vi "Insert SET ID Signal.vi"(10 "Digital Waveform Graph":digitalwaveform(graph)={"t0"=timestamp(3403282811.6192408 s since 1904-01-01), "dt"=9.615384615384615e-09, "Y"={"transitions"=[], "data"=[[1, 0, 1, 0], [1, 0, 1, 0], [1, 0, 1, 0], [1, 0, 1, 0], [1, 0, 1, 0], [1, 0, 1, 0], [1, 0, 1, 0], [0, 0, 1, 0], [0, 0, 0, 0], [0, 0, 0, 0], [0, 0, 0, 0], [0, 0, 0, 0], [0, 0, 0, 0], [0, 0, 0, 0], [0, 0, 0, 0], [1, 1, 0, 0], [1, 1, 1, 1], [1, 1, 1, 1], [1, 1, 1, 1], [1, 0, 1, 1], [1, 0, 1, 0], [1, 0, 1, 0], [1, 0, 1, 0], [1, 1, 1, 0], [1, 1, 1, 1], [1, 1, 1, 1], [1, 1, 1, 1], [1, 0, 1, 1], [1, 0, 1, 0], [1, 0, 1, 0], [1, 0, 1, 0], [1, 1, 1, 0], [1, 1, 1, 1], [1, 1, 1, 1], [1, 1, 1, 1], [1, 0, 1, 1], [1, 0, 1, 0], [1, 0, 1, 0], [1, 0, 1, 0], [1, 1, 1, 0], [1, 1, 1, 1], [1, 1, 1, 1], [1, 1, 1, 1], [1, 0, 1, 1], [1, 0, 1, 0], [1, 0, 1, 0], [1, 0, 1, 0], [0, 1, 1, 0], [0, 1, 0, 1], [0, 1, 0, 1], [0, 1, 0, 1], [0, 0, 0, 1], [0, 0, 0, 0], [0, 0, 0, 0], [0, 0, 0, 0], [1, 1, 0, 0], [1, 1, 1, 1], [1, 1, 1, 1], [1, 1, 1, 1], [1, 0, 1, 1], [1, 0, 1, 0], [1, 0, 1, 0], [1, 0, 1, 0], [0, 1, 1, 0], [0, 1, 0, 1], [0, 1, 0, 1], [0, 1, 0, 1], [0, 0, 0, 1], [0, 0, 0, 0], [0, 0, 0, 0], [0, 0, 0, 0], [1, 1, 0, 0], [1, 1, 1, 1], [1, 1, 1, 1], [1, 1, 1, 1], [1, 0, 1, 1], [1, 0, 1, 0], [1, 0, 1, 0], [1, 0, 1, 0], [1, 1, 1, 0], [1, 1, 1, 1], [1, 1, 1, 1], [1, 1, 1, 1], [1, 0, 1, 1], [1, 0, 1, 0], [1, 0, 1, 0], [1, 0, 1, 0], [0, 1, 1, 0], [0, 1, 0, 1], [0, 1, 0, 1], [0, 1, 0, 1], [0, 0, 0, 1], [0, 0, 0, 0], [0, 0, 0, 0], [0, 0, 0, 0], [1, 1, 0, 0], [1, 1, 1, 1], [1, 1, 1, 1], [1, 1, 1, 1], [1, 0, 1, 1], [1, 0, 1, 0], [1, 0, 1, 0], [1, 0, 1, 0], [0, 1, 1, 0], [0, 1, 0, 1], [0, 1, 0, 1], [0, 1, 0, 1], [0, 0, 0, 1], [0, 0, 0, 0], [0, 0, 0, 0], [0, 0, 0, 0], [1, 1, 0, 0], [1, 1, 1, 1], [1, 1, 1, 1], [1, 1, 1, 1], [1, 0, 1, 1], [1, 0, 1, 0], [1, 0, 1, 0], [1, 0, 1, 0], [0, 1, 1, 0], [0, 1, 0, 1], [0, 1, 0, 1], [0, 1, 0, 1], [0, 0, 0, 1], [0, 0, 0, 0], [0, 0, 0, 0], [0, 0, 0, 0], [0, 1, 0, 0], [0, 1, 0, 1], [0, 1, 0, 1], [0, 1, 0, 1], [0, 0, 0, 1], [0, 0, 0, 0], [0, 0, 0, 0], [0, 0, 0, 0], [0, 1, 0, 0], [0, 1, 0, 1], [0, 1, 0, 1], [0, 1, 0, 1], [0, 0, 0, 1], [0, 0, 0, 0], [0, 0, 0, 0], [0, 0, 0, 0], [0, 1, 0, 0], [0, 1, 0, 1], [0, 1, 0, 1], [0, 1, 0, 1], [0, 0, 0, 1], [0, 0, 0, 0], [0, 0, 0, 0], [0, 0, 0, 0], [0, 1, 0, 0], [0, 1, 0, 1], [0, 1, 0, 1], [0, 1, 0, 1], [0, 0, 0, 1], [0, 0, 0, 0], [0, 0, 0, 0], [0, 0, 0, 0], [0, 1, 0, 0], [0, 1, 0, 1], [0, 1, 0, 1], [0, 1, 0, 1], [0, 0, 0, 1], [0, 0, 0, 0], [0, 0, 0, 0], [0, 0, 0, 0], [0, 1, 0, 0], [0, 1, 0, 1], [0, 1, 0, 1], [0, 1, 0, 1], [0, 0, 0, 1], [0, 0, 0, 0], [0, 0, 0, 0], [0, 0, 0, 0], [1, 1, 0, 0], [1, 1, 1, 1], [1, 1, 1, 1], [1, 1, 1, 1], [1, 0, 1, 1], [1, 0, 1, 0], [1, 0, 1, 0], [1, 0, 1, 0], [0, 1, 1, 0], [0, 1, 0, 1], [0, 1, 0, 1], [0, 1, 0, 1], [0, 0, 0, 1], [0, 0, 0, 0], [0, 0, 0, 0], [0, 0, 0, 0], [0, 1, 0, 0], [0, 1, 0, 1], [0, 1, 0, 1], [0, 1, 0, 1], [0, 0, 0, 1], [0, 0, 0, 0], [0, 0, 0, 0], [0, 0, 0, 0], [1, 0, 0, 0], [1, 0, 1, 0], [1, 0, 1, 0], [1, 0, 1, 0], [1, 0, 1, 0], [1, 0, 1, 0], [1, 0, 1, 0], [1, 0, 1, 0], [0, 0, 1, 0], [0, 0, 0, 0], [0, 0, 0, 0], [0, 0, 0, 0], [0, 0, 0, 0], [0, 0, 0, 0], [0, 0, 0, 0], [0, 0, 0, 0], [1, 1, 0, 0], [1, 1, 1, 1], [1, 1, 1, 1], [1, 1, 1, 1], [1, 0, 1, 1], [1, 0, 1, 0], [1, 0, 1, 0], [1, 0, 1, 0], [1, 1, 1, 0], [1, 1, 1, 1], [1, 1, 1, 1], [1, 1, 1, 1], [1, 0, 1, 1], [1, 0, 1, 0], [1, 0, 1, 0], [1, 0, 1, 0], [1, 1, 1, 0], [1, 1, 1, 1], [1, 1, 1, 1], [1, 1, 1, 1], [1, 0, 1, 1], [1, 0, 1, 0], [1, 0, 1, 0], [1, 0, 1, 0], [1, 1, 1, 0], [1, 1, 1, 1], [1, 1, 1, 1], [1, 1, 1, 1], [1, 0, 1, 1], [1, 0, 1, 0], [1, 0, 1, 0], [1, 0, 1, 0], [0, 1, 1, 0], [0, 1, 0, 1], [0, 1, 0, 1], [0, 1, 0, 1], [0, 0, 0, 1], [0, 0, 0, 0], [0, 0, 0, 0], [0, 0, 0, 0], [1, 1, 0, 0], [1, 1, 1, 1], [1, 1, 1, 1], [1, 1, 1, 1], [1, 0, 1, 1], [1, 0, 1, 0], [1, 0, 1, 0], [1, 0, 1, 0], [1, 1, 1, 0], [1, 1, 1, 1], [1, 1, 1, 1], [1, 1, 1, 1], [1, 0, 1, 1], [1, 0, 1, 0], [1, 0, 1, 0], [1, 0, 1, 0], [1, 1, 1, 0], [1, 1, 1, 1], [1, 1, 1, 1], [1, 1, 1, 1], [1, 0, 1, 1], [1, 0, 1, 0], [1, 0, 1, 0], [1, 0, 1, 0], [1, 1, 1, 0], [1, 1, 1, 1], [1, 1, 1, 1], [1, 1, 1, 1], [1, 0, 1, 1], [1, 0, 1, 0], [1, 0, 1, 0], [1, 0, 1, 0], [0, 1, 1, 0], [0, 1, 0, 1], [0, 1, 0, 1], [0, 1, 0, 1], [0, 0, 0, 1], [0, 0, 0, 0], [0, 0, 0, 0], [0, 0, 0, 0], [1, 1, 0, 0], [1, 1, 1, 1], [1, 1, 1, 1], [1, 1, 1, 1], [1, 0, 1, 1], [1, 0, 1, 0], [1, 0, 1, 0], [1, 0, 1, 0], [0, 1, 1, 0], [0, 1, 0, 1], [0, 1, 0, 1], [0, 1, 0, 1], [0, 0, 0, 1], [0, 0, 0, 0], [0, 0, 0, 0], [0, 0, 0, 0], [0, 1, 0, 0], [0, 1, 0, 1], [0, 1, 0, 1], [0, 1, 0, 1], [0, 0, 0, 1], [0, 0, 0, 0], [0, 0, 0, 0], [0, 0, 0, 0], [0, 1, 0, 0], [0, 1, 0, 1], [0, 1, 0, 1], [0, 1, 0, 1], [0, 0, 0, 1], [0, 0, 0, 0], [0, 0, 0, 0], [0, 0, 0, 0], [0, 1, 0, 0], [0, 1, 5, 1], [0, 1, 5, 1], [0, 1, 5, 1], [0, 0, 5, 1], [0, 0, 4, 0], [0, 0, 5, 0], [0, 0, 5, 0], [0, 1, 5, 0], [0, 1, 5, 1], [0, 1, 5, 1], [0, 1, 5, 1], [0, 0, 5, 1], [0, 0, 3, 0], [0, 0, 5, 0], [0, 0, 5, 0], [0, 1, 5, 0], [0, 1, 5, 1], [0, 1, 5, 1], [0, 1, 5, 1], [0, 0, 5, 1], [0, 0, 4, 0], [0, 0, 5, 0], [0, 0, 5, 0], [0, 1, 5, 0], [0, 1, 5, 1], [0, 1, 5, 1], [0, 1, 5, 1], [0, 0, 5, 1], [0, 0, 3, 0], [0, 0, 5, 0], [0, 0, 5, 0], [0, 1, 5, 0], [0, 1, 5, 1], [0, 1, 5, 1], [0, 1, 5, 1], [0, 0, 5, 1], [0, 0, 4, 0], [0, 0, 5, 0], [0, 0, 5, 0], [0, 1, 5, 0], [0, 1, 5, 1], [0, 1, 5, 1], [0, 1, 5, 1], [0, 0, 5, 1], [0, 0, 3, 0], [0, 0, 5, 0], [0, 0, 5, 0], [0, 1, 5, 0], [0, 1, 5, 1], [0, 1, 5, 1], [0, 1, 5, 1], [0, 0, 5, 1], [0, 0, 4, 0], [0, 0, 5, 0], [0, 0, 5, 0], [0, 1, 5, 0], [0, 1, 5, 1], [0, 1, 5, 1], [1, 1, 5, 1], [1, 0, 5, 1], [1, 0, 3, 0], [1, 0, 5, 0], [1, 0, 5, 0], [1, 1, 5, 0], [1, 1, 5, 1], [1, 1, 5, 1], [0, 1, 5, 1], [0, 0, 5, 1], [0, 0, 4, 0], [1, 0, 5, 0], [0, 0, 5, 0], [0, 1, 5, 0], [0, 1, 0, 1], [0, 1, 0, 1], [0, 1, 0, 1], [0, 0, 0, 1], [0, 0, 0, 0], [0, 0, 0, 0], [0, 0, 0, 0], [0, 0, 0, 0]]}}, 11 "SetID_Pin_State":enum16{"0", "1", "Z"}(ring)) -> (3 "Digital Waveform Graph 2":digitalwaveform(graph)={"t0"=timestamp(3403282811.6192408 s since 1904-01-01), "dt"=9.615384615384615e-09, "Y"={"transitions"=[], "data"=[[1, 0, 1, 0], [1, 0, 1, 0], [1, 0, 1, 0], [1, 0, 1, 0], [1, 0, 1, 0], [1, 0, 1, 0], [1, 0, 1, 0], [0, 0, 1, 0], [0, 0, 0, 0], [0, 0, 0, 0], [0, 0, 0, 0], [0, 0, 0, 0], [0, 0, 0, 0], [0, 0, 0, 0], [0, 0, 0, 0], [1, 1, 0, 0], [1, 1, 1, 1], [1, 1, 1, 1], [1, 1, 1, 1], [1, 0, 1, 1], [1, 0, 1, 0], [1, 0, 1, 0], [1, 0, 1, 0], [1, 1, 1, 0], [1, 1, 1, 1], [1, 1, 1, 1], [1, 1, 1, 1], [1, 0, 1, 1], [1, 0, 1, 0], [1, 0, 1, 0], [1, 0, 1, 0], [1, 1, 1, 0], [1, 1, 1, 1], [1, 1, 1, 1], [1, 1, 1, 1], [1, 0, 1, 1], [1, 0, 1, 0], [1, 0, 1, 0], [1, 0, 1, 0], [1, 1, 1, 0], [1, 1, 1, 1], [1, 1, 1, 1], [1, 1, 1, 1], [1, 0, 1, 1], [1, 0, 1, 0], [1, 0, 1, 0], [1, 0, 1, 0], [0, 1, 1, 0], [0, 1, 0, 1], [0, 1, 0, 1], [0, 1, 0, 1], [0, 0, 0, 1], [0, 0, 0, 0], [0, 0, 0, 0], [0, 0, 0, 0], [1, 1, 0, 0], [1, 1, 1, 1], [1, 1, 1, 1], [1, 1, 1, 1], [1, 0, 1, 1], [1, 0, 1, 0], [1, 0, 1, 0], [1, 0, 1, 0], [0, 1, 1, 0], [0, 1, 0, 1], [0, 1, 0, 1], [0, 1, 0, 1], [0, 0, 0, 1], [0, 0, 0, 0], [0, 0, 0, 0], [0, 0, 0, 0], [1, 1, 0, 0], [1, 1, 1, 1], [1, 1, 1, 1], [1, 1, 1, 1], [1, 0, 1, 1], [1, 0, 1, 0], [1, 0, 1, 0], [1, 0, 1, 0], [1, 1, 1, 0], [1, 1, 1, 1], [1, 1, 1, 1], [1, 1, 1, 1], [1, 0, 1, 1], [1, 0, 1, 0], [1, 0, 1, 0], [1, 0, 1, 0], [0, 1, 1, 0], [0, 1, 0, 1], [0, 1, 0, 1], [0, 1, 0, 1], [0, 0, 0, 1], [0, 0, 0, 0], [0, 0, 0, 0], [0, 0, 0, 0], [1, 1, 0, 0], [1, 1, 1, 1], [1, 1, 1, 1], [1, 1, 1, 1], [1, 0, 1, 1], [1, 0, 1, 0], [1, 0, 1, 0], [1, 0, 1, 0], [0, 1, 1, 0], [0, 1, 0, 1], [0, 1, 0, 1], [0, 1, 0, 1], [0, 0, 0, 1], [0, 0, 0, 0], [0, 0, 0, 0], [0, 0, 0, 0], [1, 1, 0, 0], [1, 1, 1, 1], [1, 1, 1, 1], [1, 1, 1, 1], [1, 0, 1, 1], [1, 0, 1, 0], [1, 0, 1, 0], [1, 0, 1, 0], [0, 1, 1, 0], [0, 1, 0, 1], [0, 1, 0, 1], [0, 1, 0, 1], [0, 0, 0, 1], [0, 0, 0, 0], [0, 0, 0, 0], [0, 0, 0, 0], [0, 1, 0, 0], [0, 1, 0, 1], [0, 1, 0, 1], [0, 1, 0, 1], [0, 0, 0, 1], [0, 0, 0, 0], [0, 0, 0, 0], [0, 0, 0, 0], [0, 1, 0, 0], [0, 1, 0, 1], [0, 1, 0, 1], [0, 1, 0, 1], [0, 0, 0, 1], [0, 0, 0, 0], [0, 0, 0, 0], [0, 0, 0, 0], [0, 1, 0, 0], [0, 1, 0, 1], [0, 1, 0, 1], [0, 1, 0, 1], [0, 0, 0, 1], [0, 0, 0, 0], [0, 0, 0, 0], [0, 0, 0, 0], [0, 1, 0, 0], [0, 1, 0, 1], [0, 1, 0, 1], [0, 1, 0, 1], [0, 0, 0, 1], [0, 0, 0, 0], [0, 0, 0, 0], [0, 0, 0, 0], [0, 1, 0, 0], [0, 1, 0, 1], [0, 1, 0, 1], [0, 1, 0, 1], [0, 0, 0, 1], [0, 0, 0, 0], [0, 0, 0, 0], [0, 0, 0, 0], [0, 1, 0, 0], [0, 1, 0, 1], [0, 1, 0, 1], [0, 1, 0, 1], [0, 0, 0, 1], [0, 0, 0, 0], [0, 0, 0, 0], [0, 0, 0, 0], [1, 1, 0, 0], [1, 1, 1, 1], [1, 1, 1, 1], [1, 1, 1, 1], [1, 0, 1, 1], [1, 0, 1, 0], [1, 0, 1, 0], [1, 0, 1, 0], [0, 1, 1, 0], [0, 1, 0, 1], [0, 1, 0, 1], [0, 1, 0, 1], [0, 0, 0, 1], [0, 0, 0, 0], [0, 0, 0, 0], [0, 0, 0, 0], [0, 1, 0, 0], [0, 1, 0, 1], [0, 1, 0, 1], [0, 1, 0, 1], [0, 0, 0, 1], [0, 0, 0, 0], [0, 0, 0, 0], [0, 0, 0, 0], [1, 0, 0, 0], [1, 0, 1, 0], [1, 0, 1, 0], [1, 0, 1, 0], [1, 0, 1, 0], [1, 0, 1, 0], [1, 0, 1, 0], [1, 0, 1, 0], [0, 0, 1, 0], [0, 0, 0, 0], [0, 0, 0, 0], [0, 0, 0, 0], [0, 0, 0, 0], [0, 0, 0, 0], [0, 0, 0, 0], [0, 0, 0, 0], [1, 1, 0, 0], [1, 1, 1, 1], [1, 1, 1, 1], [1, 1, 1, 1], [1, 0, 1, 1], [1, 0, 1, 0], [1, 0, 1, 0], [1, 0, 1, 0], [1, 1, 1, 0], [1, 1, 1, 1], [1, 1, 1, 1], [1, 1, 1, 1], [1, 0, 1, 1], [1, 0, 1, 0], [1, 0, 1, 0], [1, 0, 1, 0], [1, 1, 1, 0], [1, 1, 1, 1], [1, 1, 1, 1], [1, 1, 1, 1], [1, 0, 1, 1], [1, 0, 1, 0], [1, 0, 1, 0], [1, 0, 1, 0], [1, 1, 1, 0], [1, 1, 1, 1], [1, 1, 1, 1], [1, 1, 1, 1], [1, 0, 1, 1], [1, 0, 1, 0], [1, 0, 1, 0], [1, 0, 1, 0], [0, 1, 1, 0], [0, 1, 0, 1], [0, 1, 0, 1], [0, 1, 0, 1], [0, 0, 0, 1], [0, 0, 0, 0], [0, 0, 0, 0], [0, 0, 0, 0], [1, 1, 0, 0], [1, 1, 1, 1], [1, 1, 1, 1], [1, 1, 1, 1], [1, 0, 1, 1], [1, 0, 1, 0], [1, 0, 1, 0], [1, 0, 1, 0], [1, 1, 1, 0], [1, 1, 1, 1], [1, 1, 1, 1], [1, 1, 1, 1], [1, 0, 1, 1], [1, 0, 1, 0], [1, 0, 1, 0], [1, 0, 1, 0], [1, 1, 1, 0], [1, 1, 1, 1], [1, 1, 1, 1], [1, 1, 1, 1], [1, 0, 1, 1], [1, 0, 1, 0], [1, 0, 1, 0], [1, 0, 1, 0], [1, 1, 1, 0], [1, 1, 1, 1], [1, 1, 1, 1], [1, 1, 1, 1], [1, 0, 1, 1], [1, 0, 1, 0], [1, 0, 1, 0], [1, 0, 1, 0], [0, 1, 1, 0], [0, 1, 0, 1], [0, 1, 0, 1], [0, 1, 0, 1], [0, 0, 0, 1], [0, 0, 0, 0], [0, 0, 0, 0], [0, 0, 0, 0], [1, 1, 0, 0], [1, 1, 1, 1], [1, 1, 1, 1], [1, 1, 1, 1], [1, 0, 1, 1], [1, 0, 1, 0], [1, 0, 1, 0], [1, 0, 1, 0], [0, 1, 1, 0], [0, 1, 0, 1], [0, 1, 0, 1], [0, 1, 0, 1], [0, 0, 0, 1], [0, 0, 0, 0], [0, 0, 0, 0], [0, 0, 0, 0], [0, 1, 0, 0], [0, 1, 0, 1], [0, 1, 0, 1], [0, 1, 0, 1], [0, 0, 0, 1], [0, 0, 0, 0], [0, 0, 0, 0], [0, 0, 0, 0], [0, 1, 0, 0], [0, 1, 0, 1], [0, 1, 0, 1], [0, 1, 0, 1], [0, 0, 0, 1], [0, 0, 0, 0], [0, 0, 0, 0], [0, 0, 0, 0], [0, 1, 0, 0], [0, 1, 5, 1], [0, 1, 5, 1], [0, 1, 5, 1], [0, 0, 5, 1], [0, 0, 4, 0], [0, 0, 5, 0], [0, 0, 5, 0], [0, 1, 5, 0], [0, 1, 5, 1], [0, 1, 5, 1], [0, 1, 5, 1], [0, 0, 5, 1], [0, 0, 3, 0], [0, 0, 5, 0], [0, 0, 5, 0], [0, 1, 5, 0], [0, 1, 5, 1], [0, 1, 5, 1], [0, 1, 5, 1], [0, 0, 5, 1], [0, 0, 4, 0], [0, 0, 5, 0], [0, 0, 5, 0], [0, 1, 5, 0], [0, 1, 5, 1], [0, 1, 5, 1], [0, 1, 5, 1], [0, 0, 5, 1], [0, 0, 3, 0], [0, 0, 5, 0], [0, 0, 5, 0], [0, 1, 5, 0], [0, 1, 5, 1], [0, 1, 5, 1], [0, 1, 5, 1], [0, 0, 5, 1], [0, 0, 4, 0], [0, 0, 5, 0], [0, 0, 5, 0], [0, 1, 5, 0], [0, 1, 5, 1], [0, 1, 5, 1], [0, 1, 5, 1], [0, 0, 5, 1], [0, 0, 3, 0], [0, 0, 5, 0], [0, 0, 5, 0], [0, 1, 5, 0], [0, 1, 5, 1], [0, 1, 5, 1], [0, 1, 5, 1], [0, 0, 5, 1], [0, 0, 4, 0], [0, 0, 5, 0], [0, 0, 5, 0], [0, 1, 5, 0], [0, 1, 5, 1], [0, 1, 5, 1], [1, 1, 5, 1], [1, 0, 5, 1], [1, 0, 3, 0], [1, 0, 5, 0], [1, 0, 5, 0], [1, 1, 5, 0], [1, 1, 5, 1], [1, 1, 5, 1], [0, 1, 5, 1], [0, 0, 5, 1], [0, 0, 4, 0], [1, 0, 5, 0], [0, 0, 5, 0], [0, 1, 5, 0], [0, 1, 0, 1], [0, 1, 0, 1], [0, 1, 0, 1], [0, 0, 0, 1], [0, 0, 0, 0], [0, 0, 0, 0], [0, 0, 0, 0], [0, 0, 0, 0]]}})   [LabVIEW 2013]
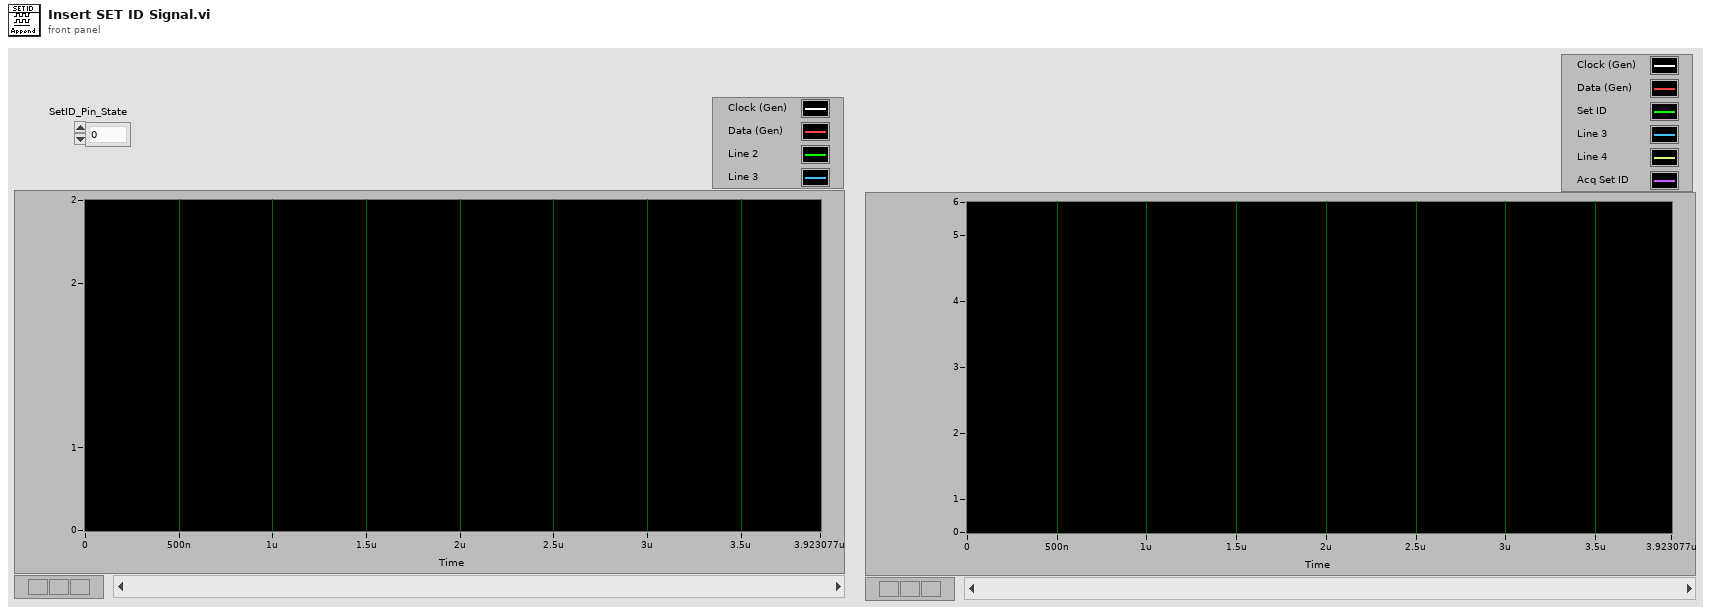
[diagram p1: front panel]
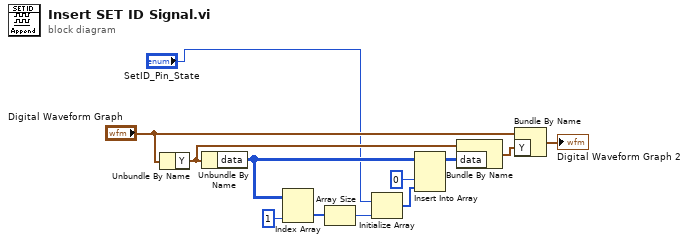
[diagram p0: block diagram]
diagram:
  n1 = Unbundle By Name("Digital Waveform Graph") -> ("Y"=w6:digitaldata)
  n2 = Unbundle By Name(w6) -> ("data"=w11:u8[][])
  n3 = Index Array(array=w11, index (col)=1 ("index (row)")) -> (element=w9:u8[])  [unwired: 1 in]
  n4 = Array Size(array=w9) -> (size(s)=w8:i32)
  n5 = Initialize Array("SetID_Pin_State", w8) -> (w7:enum16{"0", "1", "Z"}[])
  n6 = Insert Into Array(array=w11, index (col)=0 ("disabled index (col)"), new element=w7) -> (w5:u8[][])  [unwired: 1 in]
  n7 = Bundle By Name(cluster=w6, "data"=w5) -> (w4:digitaldata)
  n8 = Bundle By Name(cluster="Digital Waveform Graph", "Y"=w4) -> (→"Digital Waveform Graph 2":digitalwaveform)
